vi "PH_Timing.get Slow Trig.vi"(0 "i ref in":refnum<vi>, 5 "error in":errorcluster) -> (14 "i ref out":refnum<vi>, 19 "error out":errorcluster)   [LabVIEW 2014, in "PH_Timing.lvlib"]
doc: "This VI calculates the information concerning the slow trigger, writes them to own attributtes and publishes the information."
uses:
  PH_Timing.lvlib
  CSlibraries-extern/DimLVEvent/LVDimInterface/LVDimInterface.lvlib
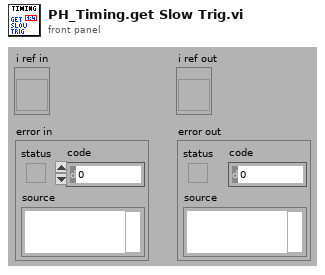
[diagram p1: front panel]
types:
  T1 = typedef "PH_Timing.lvlib/PH_Timing.i attribute.ctl" = cluster{"Sequencer":cluster{"linked?":bool, "Proc State":string, "Ref State":refnum<vi>}, "Gate Generator":cluster{"GD":cluster{"Device Status":T2, "linked?":bool}, "Settings":T3, "GUI Ref":refnum<vi>}, "Interlock Bypass":cluster{"Instancename":string, "Switch linked?":bool, "Device Status":T2, "Ref Status":refnum<vi>}, "Roughtuner":cluster{"Settings":T4, "GUI Ref":refnum<vi>, "GD":cluster{"Device Status":T2, "linked?":bool}}, "0,5Hz Gater":cluster{"Settings":T5, "GUI Ref":refnum<vi>, "GD":cluster{"Device Status":T2, "linked?":bool}}, "Slow Trigger":cluster{"Settings":T6, "GUI Ref":refnum<vi>, "Service ID Delay":i32, "Service ID Ext Trig":i32, "Wanted Settings":T6}, "Timing Mode":cluster{"Mode":T7, "GUI Ref":refnum<vi>, "Service ID T2":i32, "Service ID Mode":i32, "Wanted Mode":T7}, "ns Generator":cluster{"Settings":T8, "ns Generator Settings":refnum<vi>, "GD":cluster{"Device Status":T2, "linked?":bool}}, "Phase FEs":cluster{"Settings":T11, "GUI Ref":refnum<vi>, "Service ID Phase":i32, "Wanted Settings":T11}, "GD GUI Refs":refnum<vi>[], "Heads":T12[], "GUI Ref Delete":refnum<vi>}
  T2 = typedef "PH_StatusHandler.lvlib/PH_StatusHandler.Status.ctl" = i16
  T3 = typedef "PH_Timing.lvlib/PH_Timing.GateGen.ctl" = cluster{"Instance":string, "Channel Gate":i32, "Channel T2":i32, "Width Gate":dbl, "Width T2":dbl, "Delay Gate":dbl, "Delay T2":dbl, "Gate activ":bool, "T2 activ":bool, "System Mode":enum16{"Normal", "Single", "Burst", "Duty Cycle"}}
  T4 = typedef "PH_Timing.lvlib/PH_Timing.Roughtuner.ctl" = cluster{"Instance":string, "Phase PHELIX / UNILAC":cluster{"Channel":u16, "relative to":u16, "Delay [ms]":dbl}, "Pulse Length":cluster{"Channel":u16, "relative to":u16, "Delay [ms]":dbl}, "Trigger":cluster{"externally?":bool, "Rate [Hz]":dbl}}
  T5 = typedef "PH_Timing.lvlib/PH_Timing.0.5HzGater.ctl" = cluster{"Instance":string, "Channel ns FE Delay":i32, "Channel 0.5Hz":i32, "Width ns FE Delay":dbl, "Width 0.5Hz":dbl, "Delay ns FE Delay":dbl, "Delay 0.5Hz":dbl, "ns FE Delay active":bool, "0.5Hz activ":bool, "ns FE Delay inverted":bool, "0.5Hz inverted":bool}
  T6 = typedef "PH_Timing.lvlib/PH_Timing.Slow Trigger Settings.ctl" = cluster{"Delay":dbl, "externally triggered?":bool}
  T7 = typedef "PH_Timing.lvlib/PH_Timing.Timing Mode.ctl" = cluster{"T2":i16, "Modeselector":enum32{"10 Hz", "0.5 Hz", "Shot"}}
  T8 = typedef "PH_Timing.lvlib/PH_Timing.ns Generator.ctl" = cluster{"Instance":string, "Phase fs / ns FE":cluster{"Channel":T9, "Settings":T10}}
  T9 = typedef "Stanford Research DG645 - Driver.lvlib/Channel.ctl" = i32
  T10 = typedef "PH_SRDG645.lvlib/PH_SRDG645.Channel Settings.ctl" = cluster{"Delay [s]":dbl, "relative to":i32}
  T11 = typedef "PH_Timing.lvlib/PH_Timing.Phase FEs.ctl" = cluster{"Phase":dbl}
  T12 = typedef "PH_Timing.lvlib/PH_Timing.PU Data.ctl" = cluster{"linked?":bool, "Data":T13, "GD":cluster{"Device Status":T2, "linked?":bool}, "GUI Ref":refnum<vi>, "PU":T14}
  T13 = typedef "PH_Timing.lvlib/PH_Timing.PU Info.ctl" = cluster{"Act CH?":bool, "GD":string, "CH":i32, "Delay":dbl, "active":bool, "in Use?":bool}
  T14 = typedef "PH_PP_Common.lvlib/PH_PP_Common.PUs.ctl" = enum16{"no Info", "PA-19mm-1", "PA-19mm-2", "PA-45mm-PILC", "PA-45mm-MAIN", "MA-PU-1", "MA-PU-2", "MA-PU-3", "MA-PU-4", "MA-PU-5", "MA-PU-6", "MA-FR", "MA-PILC", "PA-45mm-DP"}
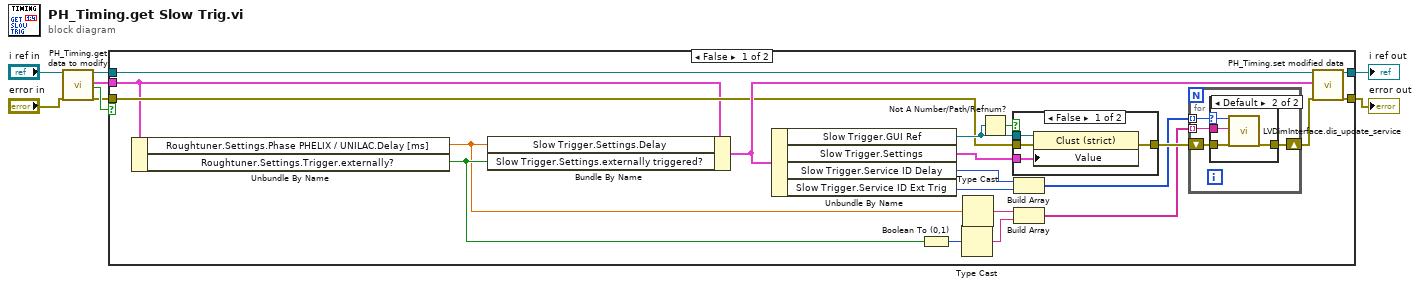
[diagram p0: block diagram]
diagram:
  n1 = call "PH_Timing.get data to modify.vi"("i ref in"="i ref in", "error in (no error)"="error in") -> ("i ref out"=w2:refnum<vi>, "i attribute"=w7:T1, "timed out"=w8:bool, "error out"=w5:errorcluster)  [unwired: 14 in]
  n2 = case shown="False" w8 {
    tunnel: w2 -> [w28 w44]
    tunnel: [w27 w44] -> w3
    tunnel: w5 -> [w20 w43]
    tunnel: [w26 w43] -> w6
    tunnel: w7 -> [w19 _]
    frame False {
      n3 = Unbundle By Name(w19) -> ("Roughtuner.Settings.Phase PHELIX / UNILAC.Delay [ms]"=w11:dbl, "Roughtuner.Settings.Trigger.externally?"=w18:bool)
      n4 = Bundle By Name(cluster=w19, "Slow Trigger.Settings.Delay"=w11, "Slow Trigger.Settings.externally triggered?"=w18) -> (w25:T1)
      n5 = Unbundle By Name(w25) -> ("Slow Trigger.GUI Ref"=w23:refnum<vi>, "Slow Trigger.Settings"=w22:T6, "Slow Trigger.Service ID Delay"=w17:i32, "Slow Trigger.Service ID Ext Trig"=w16:i32)
      n6 = Boolean To (0,1)(Boolean=w18) -> (0, 1=w15:i16)
      n7 = Type Cast(x=w15) -> (*(type *) &x=w13:string)  [unwired: 1 in]
      n8 = Type Cast(x=w11) -> (*(type *) &x=w14:string)  [unwired: 1 in]
      n9 = Not A Number/Path/Refnum?(number/path/refnum=w23) -> (NaN/Path/Refnum?=w24:bool)
      n10 = case shown="False" w24 {
        tunnel: [w41 w42] -> w21
        tunnel: w23 -> [w40 _]
        tunnel: w22 -> [w39 _]
        tunnel: w20 -> [w38 w42]
        frame False {
          n11 = property class="Clust (strict)"(reference=w40, error in=w38, "Value"=w39) -> (error out=w41:errorcluster)  [unwired: 1 out]
        }
        frame True {
        }
      }
      n12 = Build Array(w17, w16) -> (w9:i32[])
      n13 = Build Array(w14, w13) -> (w10:string[])
      n14 = for {
        tunnel: w9 -> [w31] mode=indexing
        tunnel: w10 -> [w29] mode=indexing
        shift-right: [w30] -> w12
        shift-left: w21 -> [w32]
        n15 = case shown="Default" w31 {
          selector: w31 -> [_ w35]
          tunnel: [w33 w36] -> w30
          tunnel: w32 -> [w33 w37]
          tunnel: w29 -> [_ w34]
          frame -1 {
          }
          frame Default {
            n16 = call "LVDimInterface.dis_update_service.vi"("my_serviceID"=w35, "data"=w34, "error in (no error)"=w37) -> ("error out"=w36:errorcluster)  [unwired: 14 in, 2 out]
          }
        }
      }
      n17 = call "PH_Timing.set modified data.vi"("i ref in"=w28, "i attribute"=w25, "error in (no error)"=w12) -> ("i ref out"=w27:refnum<vi>, "error out"=w26:errorcluster)  [unwired: 15 in]
    }
    frame True {
    }
  }
  "error out" <- w6
  "i ref out" <- w3
